vi "ccidinfo-w.vi"(1 "Data":string, 2 "Data Type":T1) -> ()   [LabVIEW 2013]
uses:
  Ctl/Paractl.ctl
  GlobValue.vi
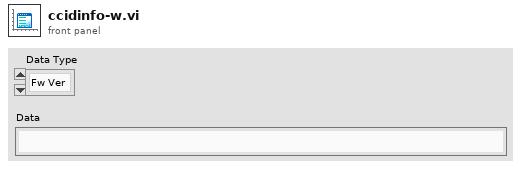
[diagram p1: front panel]
types:
  T1 = typedef "Paractl.ctl" = enum16{"Fw Ver", "HW Ver", "CCID", "WiFiName", "DevID", "SN", "TUID", "CertifID", "PdTime", "Provider", "WiFiPassword", "Imei", "AuthCode", "Reserved1", "Reserved2", "Reserved3"}
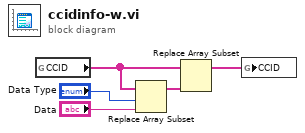
[diagram p0: block diagram]
diagram:
  n1 = global read "GlobValue.vi" "CCID"() -> (w2:string[])
  n2 = Replace Array Subset(array=w2, new element="Data", index="Data Type") -> (w4:string[])
  n3 = Replace Array Subset(array=w2, new element=w4) -> (w1:string[])  [unwired: 1 in]
  n4 = global write "GlobValue.vi" "CCID"(w1) -> ()
